vi "time elapsed.vi"() -> (3 "time elapsed since last call (in ms)":u32)   [LabVIEW 2012]
uses:
  GFG/GFGnumericGet.vi
  GFG/GFG library.lvlib
panel:
  out "Numeric":dbl
  out "x/y":dbl
  in  "avg of":dbl
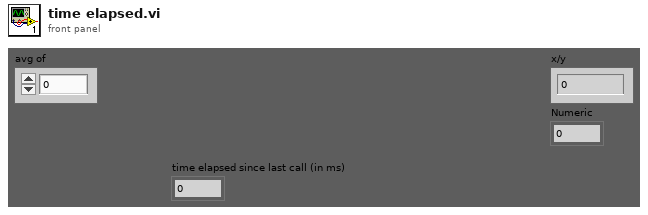
[diagram p1: front panel]
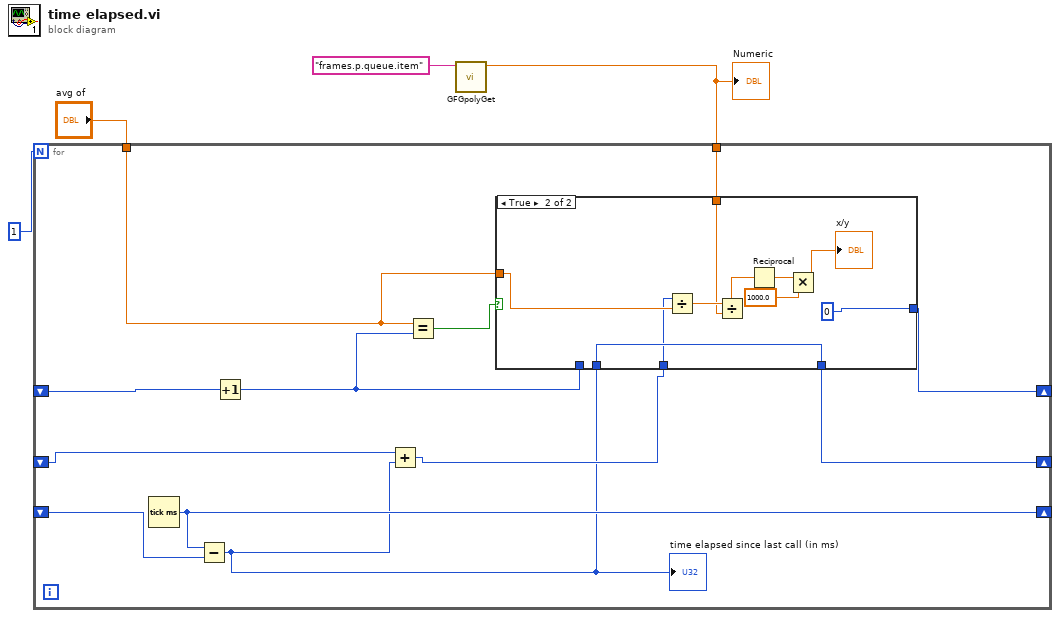
[diagram p0: block diagram]
diagram:
  n1 = call-poly "GFGpolyGet.vi"("Variable Name in"="frames.p.queue.item" ("Tag in")) -> ("Numeric"=w1:dbl)  [unwired: 9 in, 1 out]
  "Numeric" <- w1
  n2 = for {
    N: 1 -> [_]
    shift-right: [w16] -> _
    shift-left: _ -> [w15]
    shift-right: [w9] -> _
    shift-left: _ -> [w14]
    shift-right: [w11] -> _
    shift-left: _ -> [w13]
    tunnel: "avg of" -> [w6]
    tunnel: w1 -> [w5]
    n3 = Tick Count (ms)() -> (millisecond timer value=w16:u32)
    n4 = Subtract(x=w16, y=w15) -> (x-y=w7:u32)
    "time elapsed since last call (in ms)" <- w7
    n5 = Increment(x=w13) -> (x+1=w8:u32)
    n6 = Add(x=w14, y=w7) -> (x+y=w10:u32)
    n7 = Equal?(x=w6, y=w8) -> (x = y?=w12:bool)
    n8 = case shown="True" w12 {
      tunnel: [w17 u32 0] -> w11
      tunnel: w10 -> [w18 w25]
      tunnel: [w18 w27] -> w9
      tunnel: w8 -> [w17 _]
      tunnel: w7 -> [_ w27]
      tunnel: w6 -> [_ w26]
      tunnel: w5 -> [_ w19]
      frame False {
      }
      frame True {
        n9 = Divide(x=w25, y=w26) -> (x/y=w24:dbl)
        n10 = Divide(x=w24, y=w19) -> (x/y=w23:dbl)
        n11 = Reciprocal(x=w23) -> (1/x=w22:dbl)
        n12 = Multiply(x=w22, y=1000.0) -> (x*y=→"x/y":dbl)
      }
    }
  }
